vi "Close MeasurementLink Session.vi"(8 "error in":errorcluster, 9 "initialize and close session behavior":T1, 10 "session in":variant, 11 "session factory in":refnum<class "Session Factory.lvclass">) -> (0 "error out":errorcluster)   [LabVIEW 2020, in "MeasurementLink VISA.lvlib" / "Session Factory.lvclass"]
uses:
  Session Factory.lvclass
  MeasurementLink Instrument/ISession Factory/Initialize and Close Session Behavior.ctl
  Session Factory.lvclass/Session Factory.ctl
  MeasurementLink Instrument/ISession Factory/ISession Factory.lvclass
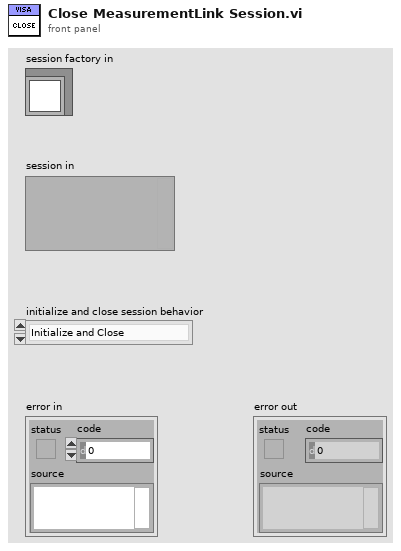
[diagram p1: front panel]
types:
  T1 = typedef "MeasurementLink Instrument.lvlib/ISession Factory.lvclass/Initialize and Close Session Behavior.ctl" = enum16{"Initialize and Close", "Attach and Detach", "Initialize and Detach", "Attach and Close"}
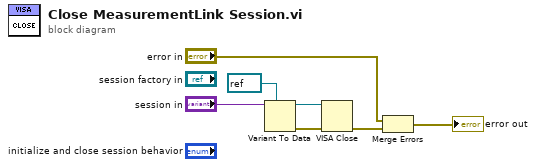
[diagram p0: block diagram]
diagram:
  n1 = Variant To Data(type=refnum<visa-resource-name> refnum ("VISA resource name out"), Variant="session in") -> (data=w4:refnum<visa-resource-name>, error out=w3:errorcluster)  [unwired: 1 in]
  n2 = VISA Close(VISA resource name=w4, error in (no error)=w3) -> (error out=w2:errorcluster)
  n3 = Merge Errors("error in", w2) -> (→"error out":errorcluster)
